vi "deviceStatusRequest.vi"(8 "error in (no error)":errorcluster, 11 "Electrometer in":refnum<class "Electrometer.lvclass">) -> (0 "error out":errorcluster, 1 "Device Code":i32[](array[numeric]), 2 "Error Message":string, 3 "Electrometer out":refnum<class "Electrometer.lvclass">)   [LabVIEW 2016, in "Electrometer.lvclass"]
uses:
  Electrometer.lvclass
  ElectrometerConfiguration/ElectrometerCOMConfiguration.lvclass
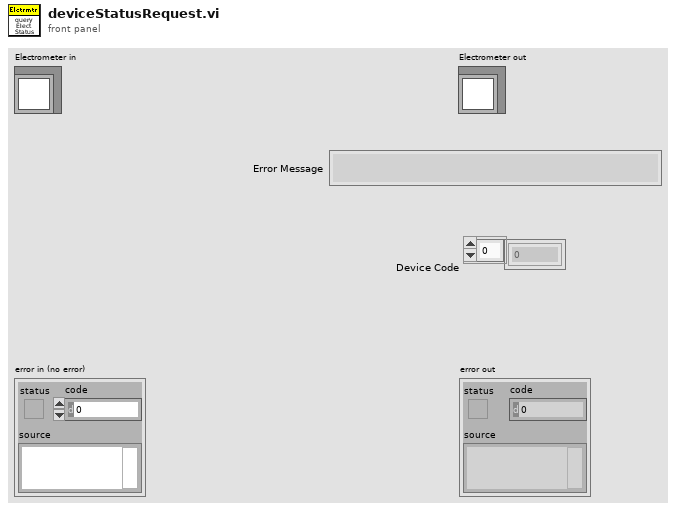
[diagram p1: front panel]
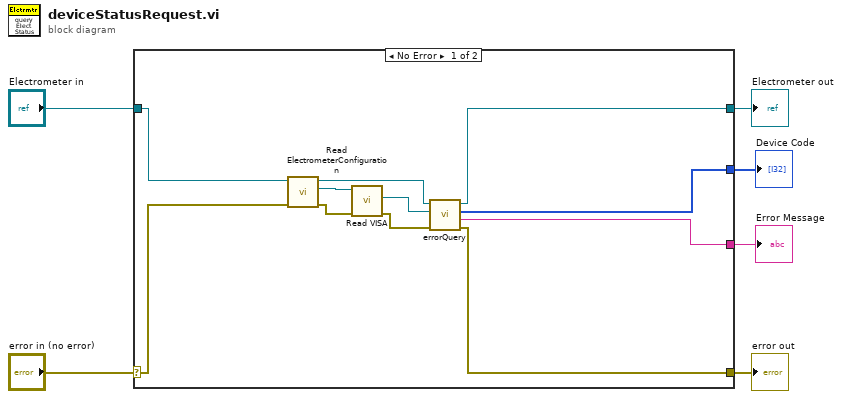
[diagram p0: block diagram]
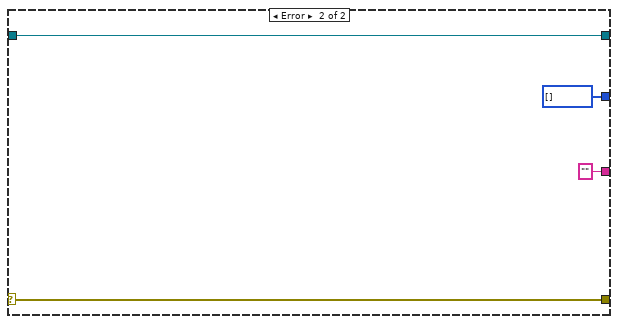
[diagram p2: hidden frame]
diagram:
  n1 = case shown="No Error" "error in (no error)" {
    selector: "error in (no error)" -> [w12 w21]
    tunnel: [w9 w21] -> w5
    tunnel: [w10 w20] -> w3
    tunnel: "Electrometer in" -> [w11 w20]
    tunnel: [w8 "" ("Error Message")] -> w2
    tunnel: [w7 i32[] [] ("Error Code")] -> w1
    frame No Error {
      n2 = call "Read ElectrometerConfiguration.vi"("error in (no error)"=w12, "Electrometer in"=w11) -> ("error out"=w14:errorcluster, "ElectrometerConfiguration"=w15:refnum<class "ElectrometerCOMConfiguration.lvclass">, "Electrometer out"=w16:refnum<class "Electrometer.lvclass">)  [unwired: 7 in]
      n3 = call-dynamic "Read VISA.vi"("error in (no error)"=w14, "ElectrometerConfiguration in"=w15) -> ("error out"=w13:errorcluster, "VISA"=w17:refnum<visa-resource-name>)  [unwired: 7 in, 1 out]
      n4 = call "errorQuery.vi"("error in (no error)"=w13, "VISA resource name"=w17, "Electrometer in"=w16) -> ("error out"=w9:errorcluster, "Error Message"=w8:string, "Device Error"=w7:i32[], "Electrometer out"=w10:refnum<class "Electrometer.lvclass">)  [unwired: 5 in]
    }
    frame Error {
    }
  }
  "error out" <- w5
  "Electrometer out" <- w3
  "Error Message" <- w2
  "Device Code" <- w1
